vi "TEST FGV User Event Reference Manager Cluster.vi"() -> (0 "Cluster":T1)   [LabVIEW 2011]
doc: "This is the Cluster for solution that tests the FGV.\n\nAAL 9/09"
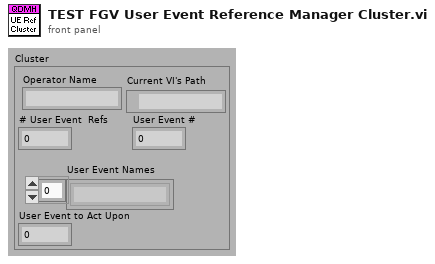
[diagram p1: front panel]
types:
  T1 = cluster{"Operator Name":string, "Current VI's Path":path, "# User Event  Refs":i32, "User Event #":i32, "User Event Names":string[], "User Event to Act Upon":i32}
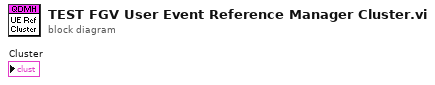
[diagram p0: block diagram]
diagram:
